vi "Test1.vi"() -> ()   [LabVIEW 2018]
panel:
  out "x+y":dbl
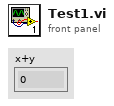
[diagram p1: front panel]
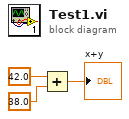
[diagram p0: block diagram]
diagram:
  n1 = Add(x=42.0, y=38.0) -> (x+y=→"x+y":dbl)
